vi "main OP300.2.vi"() -> ()   [LabVIEW 2020]
uses:
  SubVI/OP150ZP_state.ctl
  <userlib>/Alex.vi/FGV.ctl
  Lib/02 SLIM ZEN WS 500/SubVi/VG_progressBar.vi
  SubVI/CheminDeBase.vi
  VG/PN.vi
  VG/IS30%.vi
  SubVI/VG_HYDRAU.vi
  VG/VG_BT3562.vi
panel:
  out "error out":errorcluster
  in  "arrêt":bool
  in  "last?":bool
  out "VISA OUT 2":T1
  out "Cluster 2":T2
  out "IS30% ?":bool
  out "Cluster":T2
  out "progression":u8(slide) scale=0.0..100.0
  out "PN":string
  out "errout 2":errorcluster={"status"=TRUE, "code"=0, "source"="PCAN_CHANNEL ILLEGAL"} caption="errout"
  out "errout":errorcluster caption="sortie d'erreur"
  out "STOP":bool
  out "TOP":string
  out "DRAW":picture
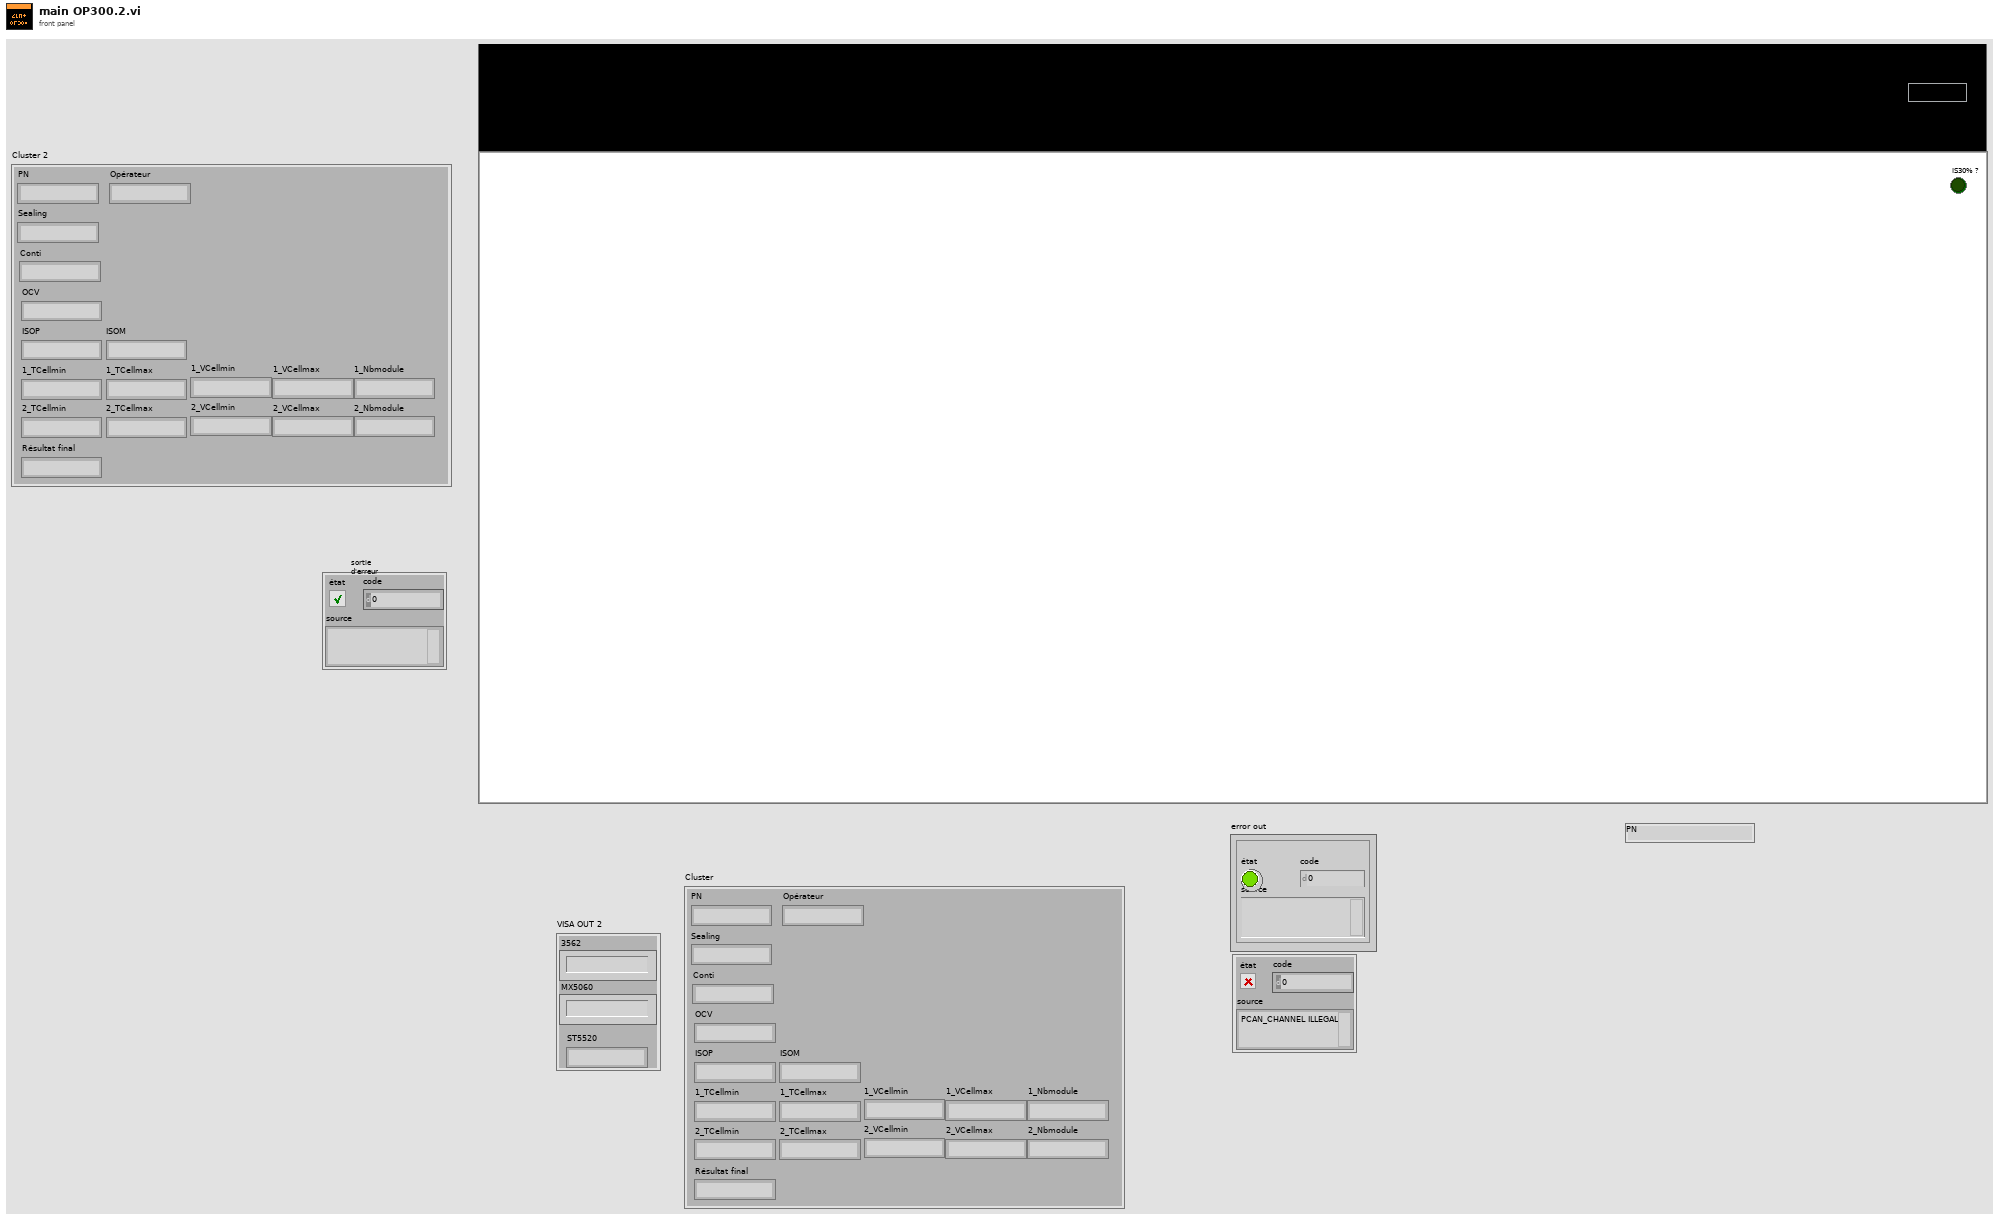
[diagram p1: front panel]
types:
  T1 = cluster{"3562":string, "MX5060":string, "ST5520":string}
  T2 = cluster{"PN":string, "Opérateur":string, "Sealing":string, "Conti":string, "OCV":string, "ISOP":string, "ISOM":string, "1_TCellmin":string, "1_TCellmax":string, "1_VCellmin":string, "1_VCellmax":string, "1_Nbmodule":string, "2_TCellmin":string, "2_TCellmax":string, "2_VCellmin":string, "2_VCellmax":string, "2_Nbmodule":string, "Résultat final":string}
  T3 = cluster{"PN":string, "Sealing":string, "Opérateur":string, "Conti":string, "OCV":string, "ISOP":string, "ISOM":string, "1_TCellmin":string, "1_TCellmax":string, "1_VCellmin":string, "1_VCellmax":string, "1_Nbmodule":string, "2_TCellmin":string, "2_TCellmax":string, "2_VCellmin":string, "2_VCellmax":string, "2_Nbmodule":string, "Résultat final":string}
  T4 = typedef "OP150ZP_state.ctl" = enum16{"Null", "Demarrage", "Init", "Scan", "Crash", "Next", "Conti", "Sealing", "Comext", ""}
  T5 = typedef "FGV.ctl" = enum16{"GET", "SET", "RAZ"}
  T6 = typedef "imagedata.ctl" = cluster{"image type":i32, "image depth":i32, "image":u8[], "mask":u8[], "colors":u32[], "Rectangle":cluster{"left":i16, "top":i16, "right":i16, "bottom":i16}}
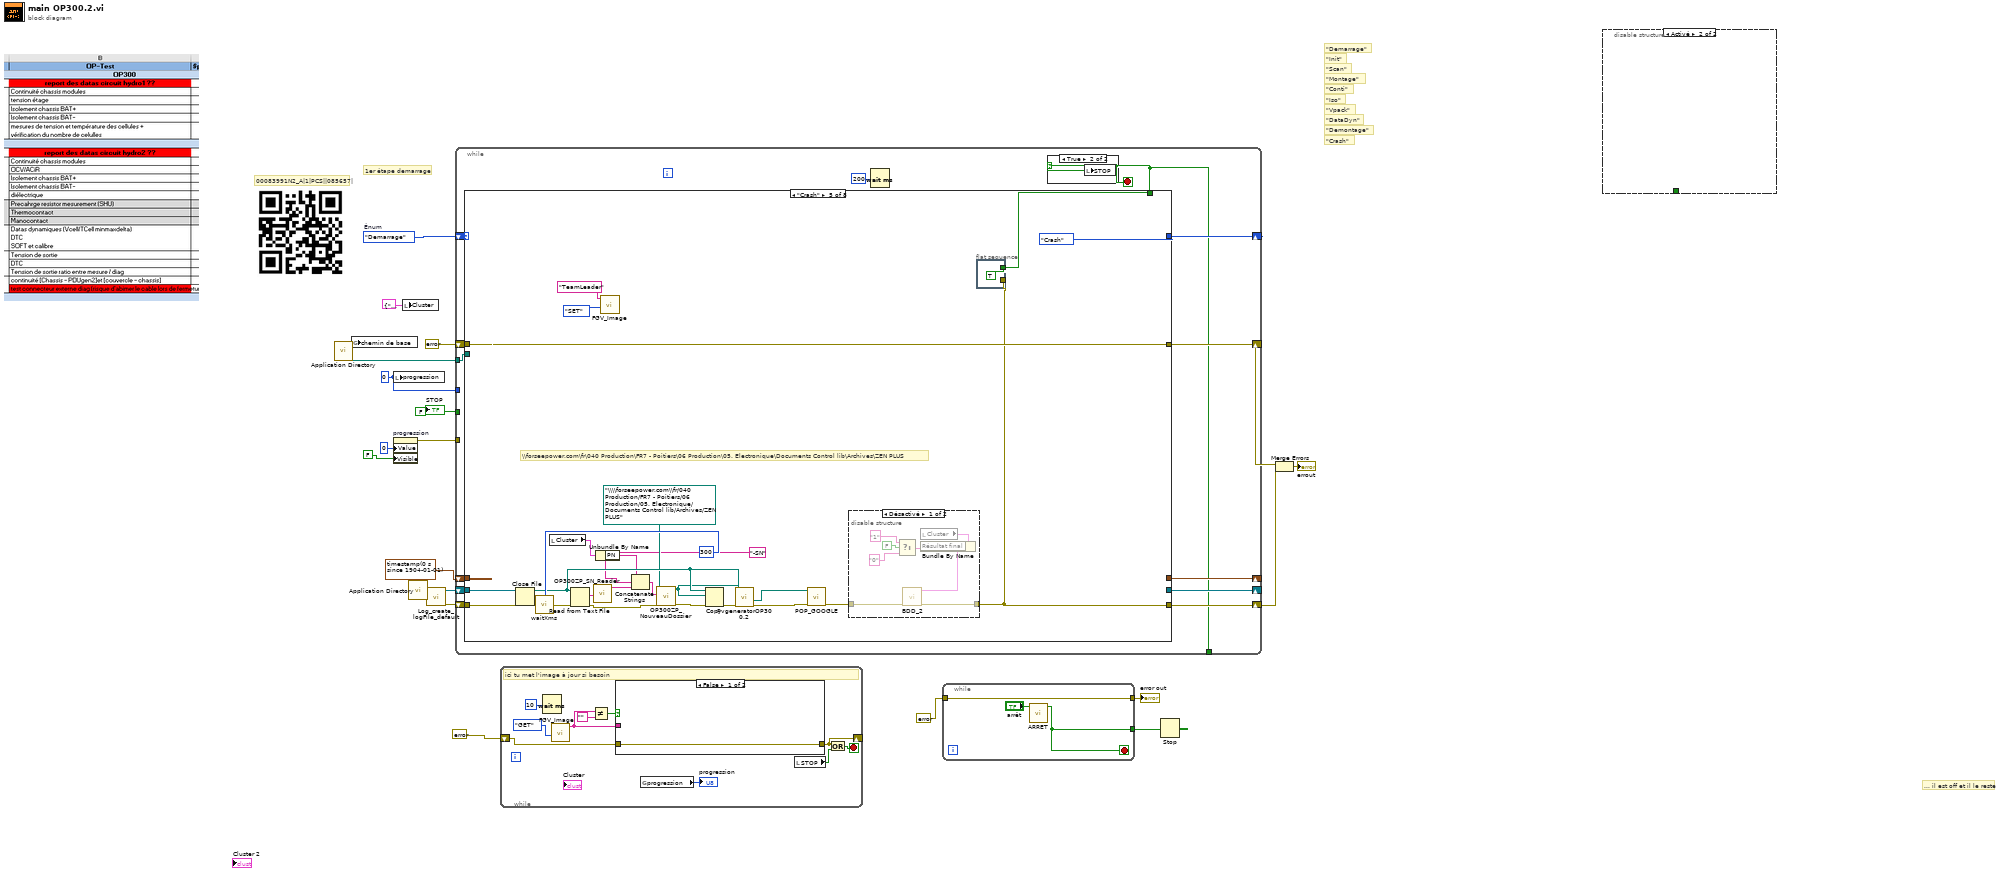
[diagram p0: block diagram]
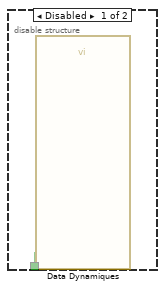
[diagram p2: hidden frame]
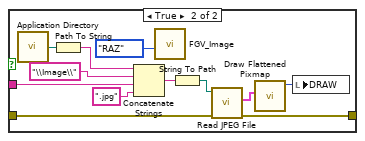
[diagram p3: hidden frame]
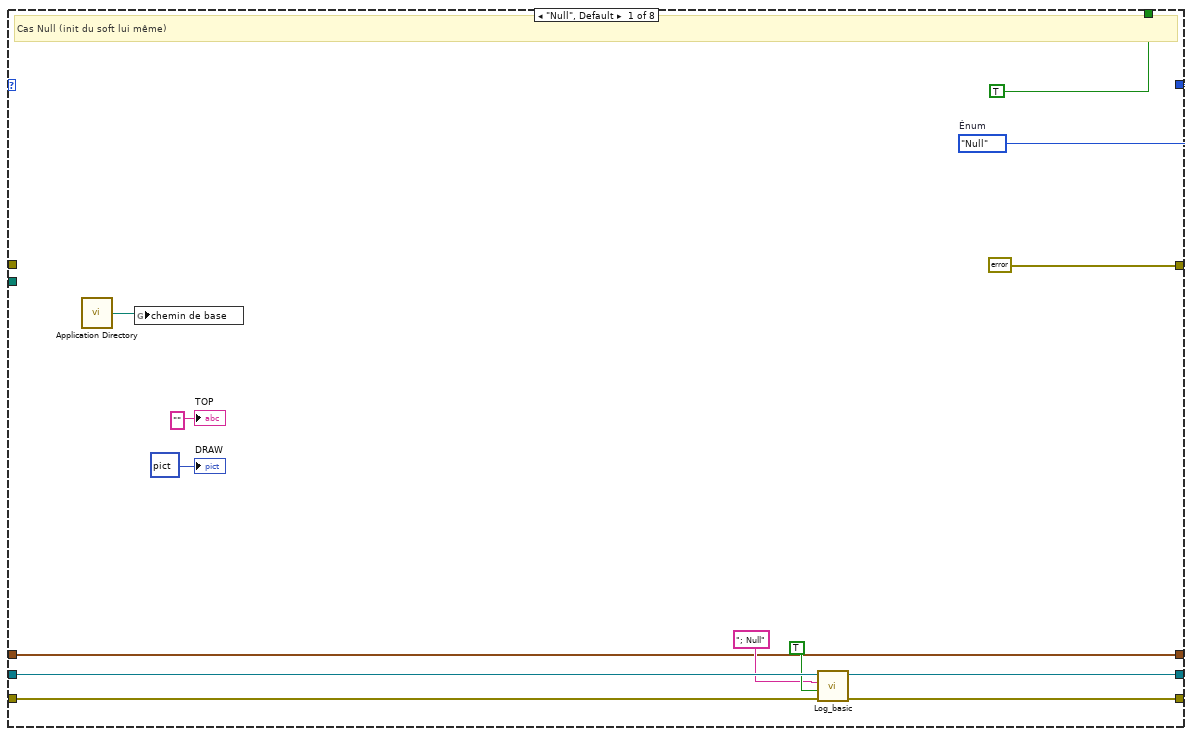
[diagram p5: hidden frame]
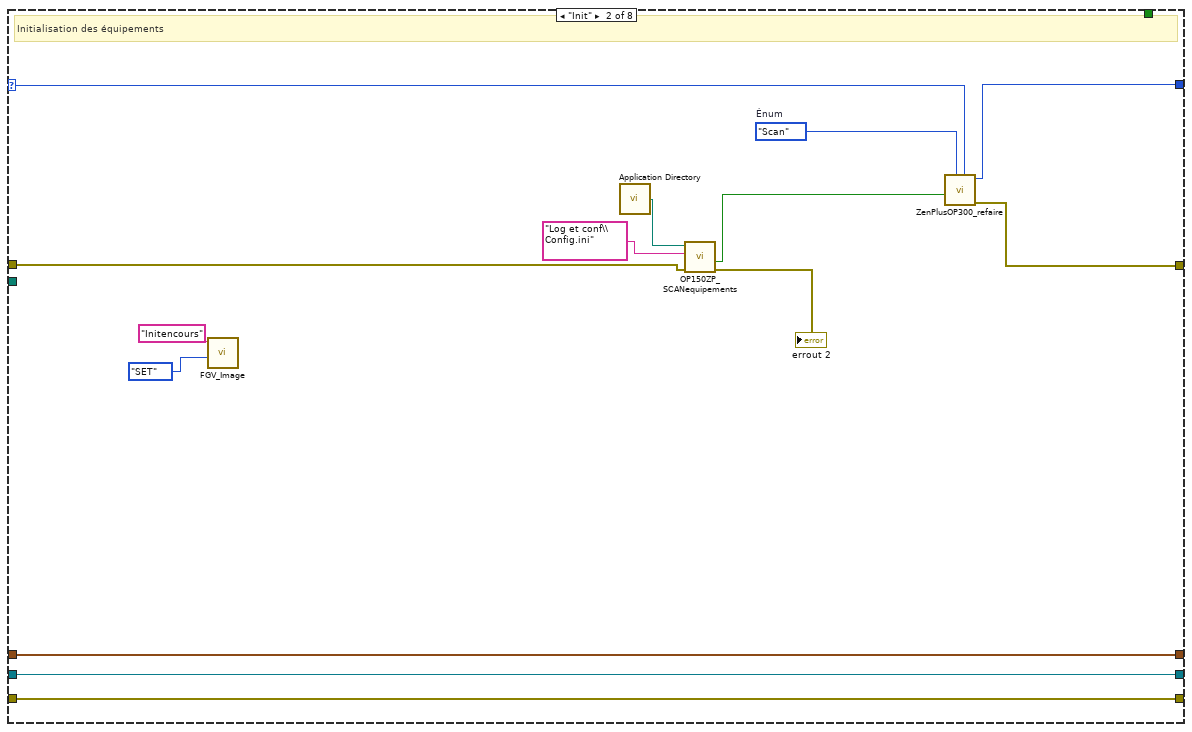
[diagram p6: hidden frame]
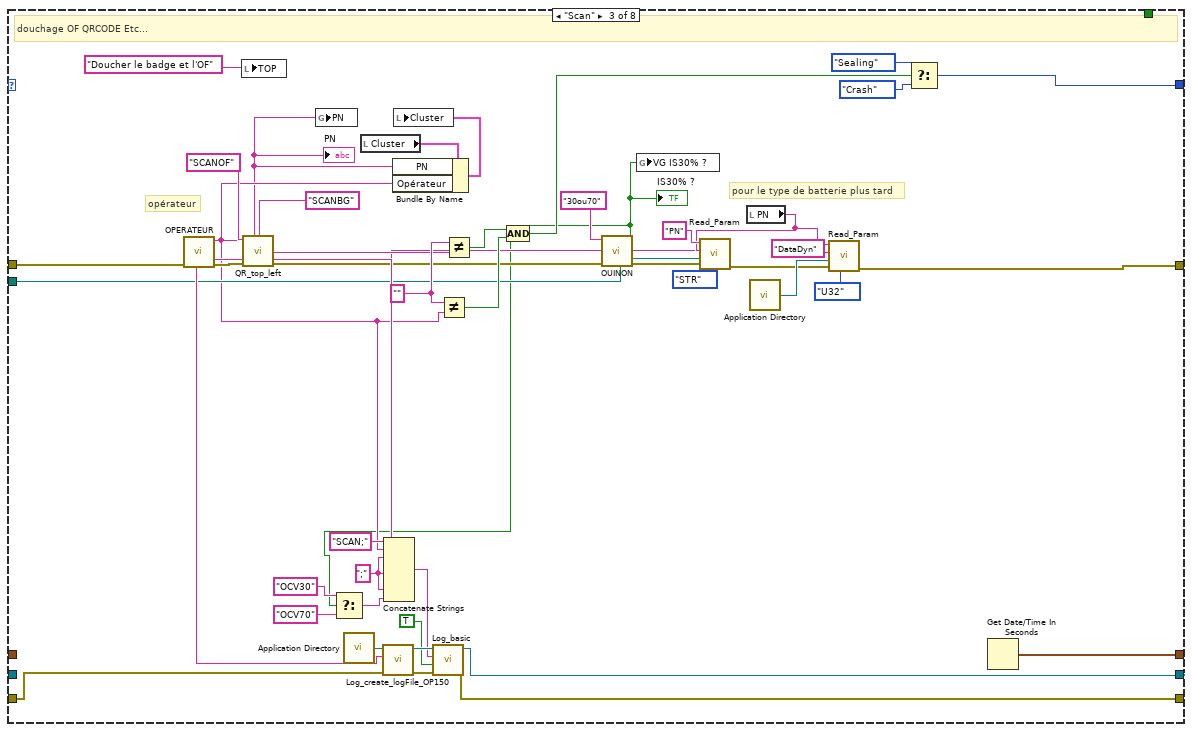
[diagram p7: hidden frame]
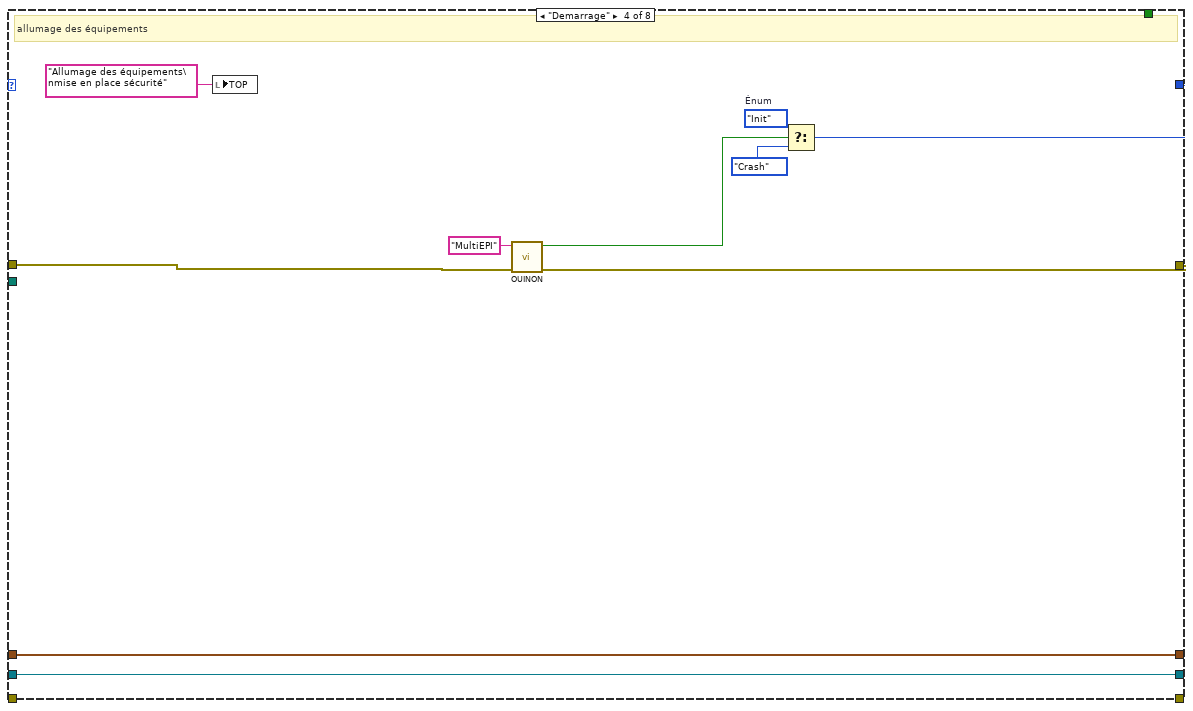
[diagram p8: hidden frame]
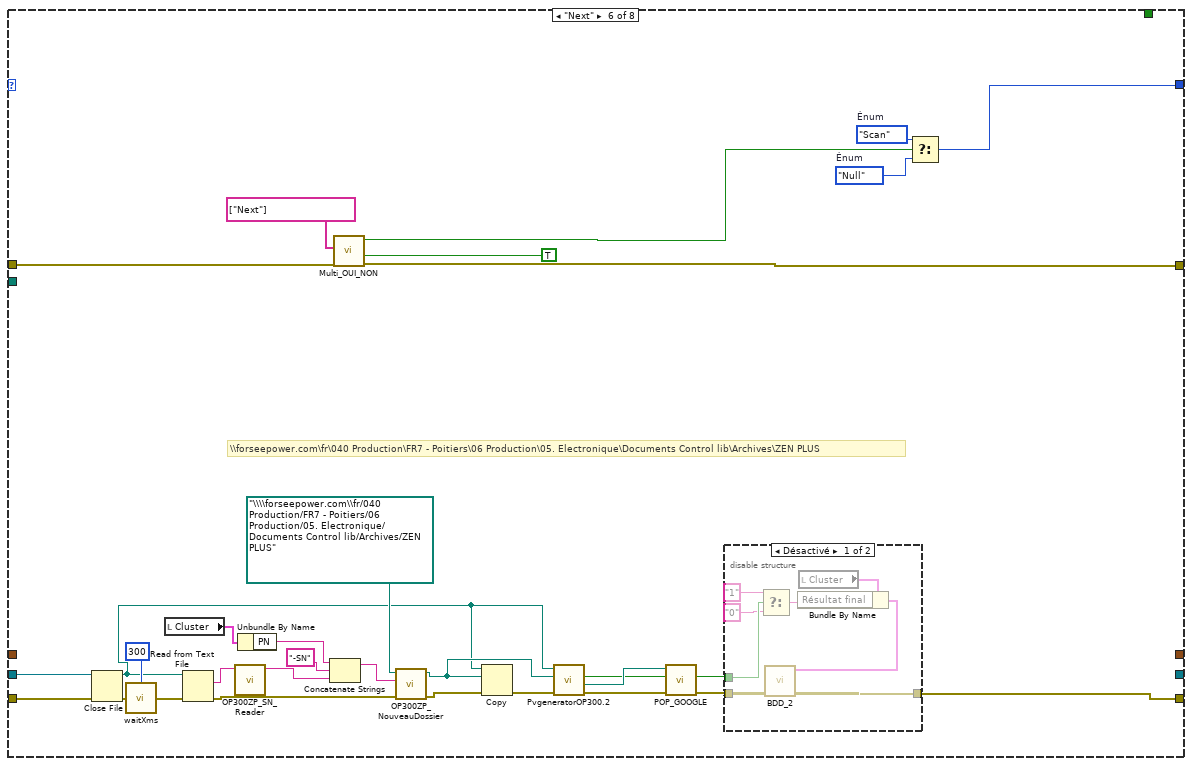
[diagram p10: hidden frame]
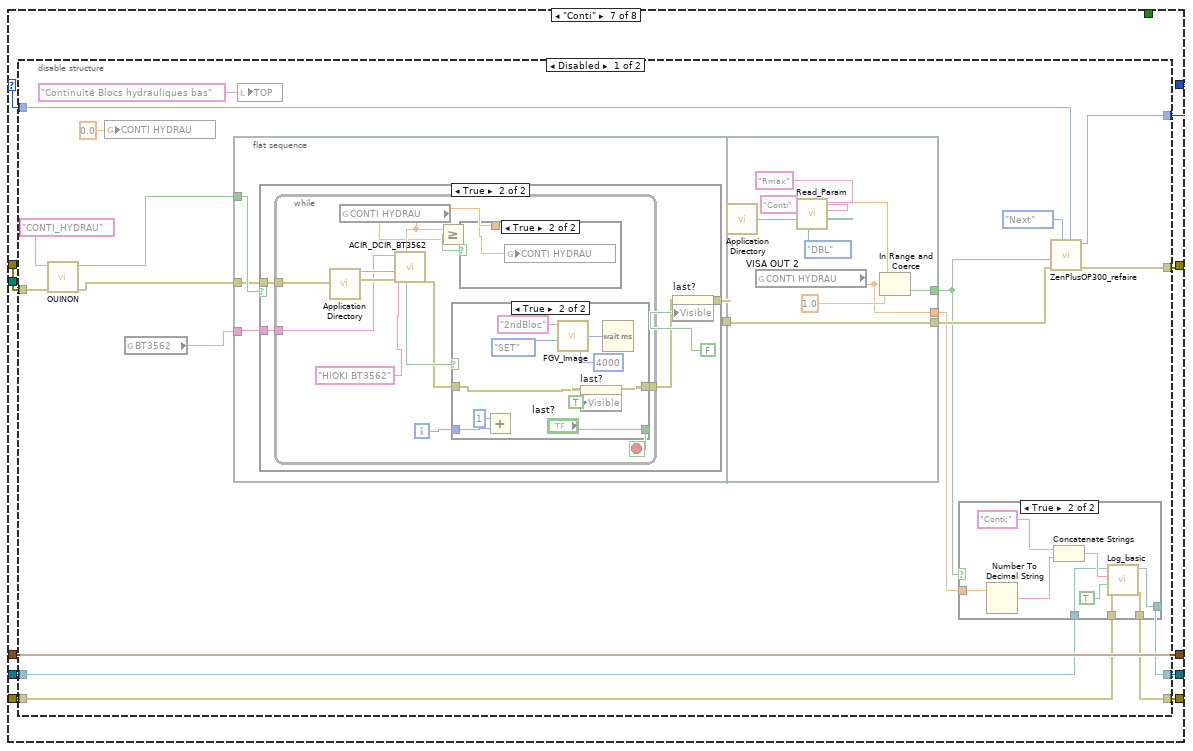
[diagram p12: hidden frame]
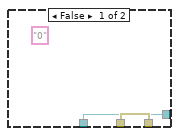
[diagram p13: hidden frame]
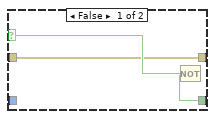
[diagram p15: hidden frame]
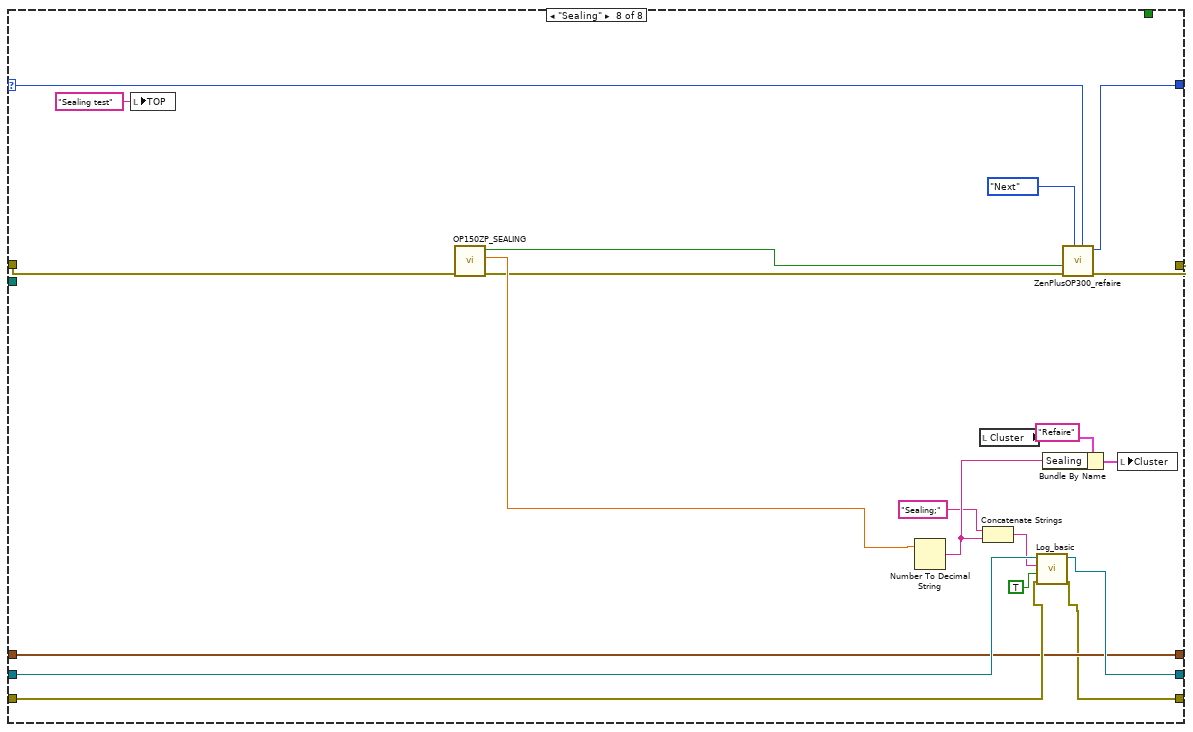
[diagram p18: hidden frame]
diagram:
  w10 = u8 0 ("progression")
  w11 = OP150ZP_state."Demarrage"  # Énum
  w17 = FALSE ("STOP")
  # "00083991N2_A|1|PCS||085657|"
  # "1er étape demarrage"
  # "\"Crash\""
  # "\"Demontage\""
  # "\"DataDyn\""
  # "\"Iso\""
  # "\"Montage\""
  # "\"Scan\""
  # "\"Init\""
  # "\"Demarrage\""
  # "\"Conti\""
  # "\"Vpack\""
  # "... il est off et il le reste"
  n1 = call <vilib>:"Application Directory.vi"() -> ("Application Directory"=w16:path)
  n2 = global write "CheminDeBase.vi" "chemin de base"(w16) -> ()
  n3 = property on="progression" class="Slide (strict)"("Value"=u8 0 ("progression"), "Visible"=FALSE) -> (error out=w8:errorcluster)  [unwired: 2 in, 1 out]
  n4 = local write "progression"(w10) -> ()
  n5 = local write "Cluster"(T3 {"PN"="0", "Sealing"="0", "Opérateur"="0", "Conti"="0", "OCV"="0", "ISOP"="0", "ISOM"="0", "1_TCellmin"="0", "1_TCellmax"="0", "1_VCellmin"="0", "1_VCellmax"="0", "1_Nbmodule"="0", "2_TCellmin"="0", "2_TCellmax"="0", "2_VCellmin"="0", "2_VCellmax"="0", "2_Nbmodule"="0", "Résultat final"="0"} ("Cluster")) -> ()
  n6 = call <vilib>:"Application Directory.vi"() -> ("Application Directory"=w14:path)
  n7 = call "Log_create_logFile_default.vi"("appdir"=w14) -> ("errout"=w15:errorcluster, "Fichier à flux d'octets en sortie"=w18:refnum<file>)  [unwired: 9 in]
  n8 = while {
    shift-right: [w32] -> w2
    shift-left: errorcluster {"status"=FALSE, "code"=0, "source"=""} ("error out") -> [w23]
    shift-right: [w22] -> _
    shift-left: w11 -> [w27]
    shift-right: [w28] -> w19
    shift-left: w15 -> [w31]
    shift-right: [w29] -> _
    shift-left: w18 -> [w30]
    tunnel: w16 -> [w26]
    tunnel: w17 -> [_]
    shift-right: [w24] -> _
    shift-left: timestamp(0 s since 1904-01-01) ("seconds since 1Jan1904") -> [w25]
    tunnel: w10 -> [_]
    tunnel: w8 -> [_]
    tunnel: [w21] -> _
    stop <- w21 stop-if-true
    n9 = case shown="\"Crash\"" w27 {
      selector: w27 -> [_ w56 _ _ _ _ w198 w282]
      tunnel: w23 -> [_ w58 w107 w109 w138 w158 w199 w280]
      tunnel: [errorcluster {"status"=FALSE, "code"=0, "source"=""} ("errin") w57 w86 w116 w138 w156 w191 w290] -> w32
      tunnel: w31 -> [w43 w61 w103 _ w141 w181 w196 w293]
      tunnel: w30 -> [w44 w60 _ w117 w142 w182 w194 w292]
      tunnel: [w41 w60 w105 w117 _ _ w193 w291] -> w29
      tunnel: [w42 w61 w106 _ w131 w174 w195 w285] -> w28
      tunnel: [TRUE _ _ _ w143 _ _ _] -> w21
      tunnel: w26 -> [_ _ w80 _ _ _ _ _]
      tunnel: w25 -> [w37 w59 _ w115 _ _ w192 w289]
      tunnel: [w37 w59 w94 w115 _ _ w192 w289] -> w24
      tunnel: [w35 w48 w62 w110 OP150ZP_state."Crash" w153 w197 w284] -> w22
      frame "Null", Default {
        w35 = OP150ZP_state."Null"  # Énum
        # "Cas Null (init du soft lui même)"
        n10 = call <vilib>:"Application Directory.vi"() -> ("Application Directory"=w47:path)
        n11 = global write "CheminDeBase.vi" "chemin de base"(w47) -> ()
        n12 = call "Log_basic.vi"("errin"=w43, "date?"=TRUE, "chaîne"="; Null", "in"=w44) -> ("sortie d'erreur"=w42:errorcluster, "refnum en sortie"=w41:refnum<file>)  [unwired: 6 in]
        "DRAW" <- picture data[5B] ("DRAW")
        "TOP" <- "" ("TOP")
      }
      frame "Init" {
        w52 = OP150ZP_state."Scan"  # Énum
        # "Initialisation des équipements"
        n13 = call <userlib>:"FGV_Image.vi"("Énum"=FGV."SET", "IN"="Initencours") -> ()  [unwired: 9 in, 1 out]
        n14 = call <vilib>:"Application Directory.vi"() -> ("Application Directory"=w49:path)
        n15 = call "OP150ZP_SCANequipements.vi"("Errin"=w58, "Chaîne"="Log et conf\\Config.ini", "pathin"=w49) -> ("ERROUT"=→"errout 2":errorcluster, "KO?"=w53:bool)  [unwired: 7 in]
        n16 = call "ZenPlusOP300_refaire.vi"("refaire"=w56, "casOK"=w52, "test ok ?"=w53) -> ("errout"=w57:errorcluster, "Next"=w48:T4)  [unwired: 7 in]
      }
      frame "Scan" {
        w66 = ";" ("chaîne")
        w97 = "" ("x")
        # "pour le type de batterie plus tard"
        # "opérateur"
        # "douchage OF QRCODE Etc..."
        n17 = call "OPERATEUR.vi"("errin"=w107, "IN"="SCANBG") -> ("error out"=w93:errorcluster, "Dataout"=w72:string)  [unwired: 8 in]
        n18 = local write "TOP"("Doucher le badge et l'OF" ("TOP")) -> ()
        n19 = call "QR_top_left.vi"("errin"=w93, "image"="SCANOF") -> ("error out"=w70:errorcluster, "Réponse"=w91:string, "SN"=w90:string, "PN"=w63:string)  [unwired: 5 in, 1 out]
        "PN" <- w63
        n20 = global write "PN.vi" "PN"(w63) -> ()
        n21 = call <vilib>:"Application Directory.vi"() -> ("Application Directory"=w104:path)
        n22 = local read "Cluster"() -> (w74:T2)
        n23 = call "Log_create_logFile_OP150.vi"("errin"=w103, "toute l'expression"=w90, "Application Directory"=w104) -> ("sortie d'erreur"=w101:errorcluster, "Fichier à flux d'octets en sortie"=w102:refnum<file>)  [unwired: 7 in]
        n24 = Bundle By Name(cluster=w74, "PN"=w63, "Opérateur"=w72) -> (w73:T2)
        n25 = local write "Cluster"(w73) -> ()
        n26 = Not Equal?(x=w97, y=w72) -> (x != y?=w95:bool)
        n27 = Not Equal?(x=w97, y=w91) -> (x != y?=w96:bool)
        n28 = Compound Arithmetic op=AND ("Opérateur arithmétique")(w96, w95) -> (w78:bool)
        n29 = call "OUINON.vi"("errin"=w70, "image"="30ou70") -> ("error out"=w69:errorcluster, "OUI/NON"=w64:bool)  [unwired: 8 in]
        "IS30% ?" <- w64
        n30 = Select ("Sélectionner")(t="OCV30" ("section"), s=w64, f="OCV70" ("section")) -> (s? t:f=w65:string)
        n31 = global write "IS30%.vi" "VG IS30% ?"(w64) -> ()
        n32 = local read "PN"() -> (w82:string)
        n33 = call "Read_Param.vi"("Énum"=enum16{"STR", "DBL", "U32"}."STR", "errin"=w69, "pathin"=w80, "section"=w82, "key"="PN") -> ("error out"=w85:errorcluster, "str"=w81:string)  [unwired: 2 in, 3 out]
        n34 = Concatenate Strings("SCAN;" ("chaîne"), w72, w66, w90, w66, w81, w66, w65) -> (w99:string)
        n35 = call "Log_basic.vi"("errin"=w101, "date?"=TRUE, "chaîne"=w99, "in"=w102) -> ("sortie d'erreur"=w106:errorcluster, "refnum en sortie"=w105:refnum<file>)  [unwired: 6 in]
        n36 = call <vilib>:"Application Directory.vi"() -> ("Application Directory"=w89:path)
        n37 = call "Read_Param.vi"("Énum"=enum16{"STR", "DBL", "U32"}."U32", "errin"=w85, "pathin"=w89, "section"="DataDyn", "key"=w82) -> ("error out"=w86:errorcluster)  [unwired: 2 in, 4 out]
        n38 = Select ("Sélectionner")(t=OP150ZP_state."Sealing" ("Énum"), s=w78, f=OP150ZP_state."Crash" ("cas faux")) -> (s? t:f=w62:T4)
        n39 = Get Date/Time In Seconds() -> (seconds since 1Jan1904=w94:timestamp)
      }
      frame "Demarrage" {
        w112 = OP150ZP_state."Init"  # Énum
        # "allumage des équipements"
        n40 = local write "TOP"("Allumage des équipements\nmise en place sécurité" ("TOP")) -> ()
        n41 = call "OUINON.vi"("errin"=w109, "image"="MultiEPI" ("IN")) -> ("error out"=w116:errorcluster, "OUI/NON"=w113:bool)  [unwired: 8 in]
        n42 = Select ("Sélectionner")(t=w112, s=w113, f=OP150ZP_state."Crash" ("cas faux")) -> (s? t:f=w110:T4)
      }
      frame "Crash" {
        # "\\\\forseepower.com\\fr\\040 Production\\FR7 - Poitiers\\06 Production\\05. Electronique\\Documents Control lib\\Archives\\ZEN PLUS"
        n43 = Close File(refnum=w142, error in=w141) -> (path=w129:path, error out=w134:errorcluster)
        n44 = call <userlib>:"waitXms.vi"("attente (ms)"=u32 300, "errin"=w134) -> ("errout"=w130:errorcluster)  [unwired: 13 in]
        n45 = local read "Cluster"() -> (w123:T2)
        n46 = Read from Text File(file (use dialog)=w129, error in=w130) -> (text=w128:string, error out=w126:errorcluster)  [unwired: 2 in, 2 out]
        n47 = call "OP300ZP_SN_Reader.vi"("Fichier txt"=w128) -> ("SN"=w121:string)  [unwired: 10 in]
        n48 = Unbundle By Name(w123) -> ("PN"=w120:string)
        n49 = call <userlib>:"FGV_Image.vi"("Énum"=FGV."SET", "IN"="TeamLeader") -> ()  [unwired: 9 in, 1 out]
        n50 = Concatenate Strings(w120, "-SN" ("chaîne"), w121) -> (w122:string)
        n51 = call "OP300ZP_NouveauDossier.vi"("entrée d'erreur (pas d'erreur)"=w126, "Nom du repertoire (PN SN)"=w122, "Network before adding a new folder"=path "\\\\forseepower.com\\fr/040 Production/FR7 - Poitiers/06 Production/05. Electronique/Documents Control lib/Archives/ZEN PLUS" ("chemin de la cible (utiliser une boîte de dialogue)")) -> ("sortie d'erreur"=w127:errorcluster, "Network after adding a new folder"=w124:path)  [unwired: 7 in]
        n52 = Copy ("Copier")(8:w127, 10:w124, 11:w129) -> (0:w133:errorcluster)  [unwired: 2 in, 2 out]
        n53 = call "PvgeneratorOP300.2.vi"("errin"=w133, "network"=w124, "path in"=w129) -> ("sortie d'erreur"=w137:errorcluster, "network out"=w136:path)  [unwired: 5 in, 2 out]
        n54 = call "POP_GOOGLE.vi"("error in"=w137, "chemin"=w136) -> ("error out"=w132:errorcluster)  [unwired: 8 in, 1 out]
        n55 = disable-structure shown="Désactivé" {
          disable-tunnel: w132 -> [w151 _]
          disable-tunnel: [w150 _] -> w131
          frame Disabled {
            n56 = Select ("Sélectionner")(t="1", s=FALSE ("sélecteur"), f="0" ("cas faux")) -> (s? t:f=w146:string)
            n57 = local read "Cluster"() -> (w149:T2)
            n58 = Bundle By Name(cluster=w149, "Résultat final"=w146) -> (w145:T2)
            n59 = call "BDD_2.vi"("errin"=w151, "Cluster"=w145) -> ("error out"=w150:errorcluster)  [unwired: 8 in, 1 out]
          }
          frame Enabled {
          }
        }
        n60 = flat-sequence {
          tunnel: [TRUE] -> w143
          tunnel: w131 -> [_]
          frame #0 {
          }
        }
      }
      frame "Next" {
        w179 = OP150ZP_state."Null"  # Énum
        w180 = OP150ZP_state."Scan"  # Énum
        # "\\\\forseepower.com\\fr\\040 Production\\FR7 - Poitiers\\06 Production\\05. Electronique\\Documents Control lib\\Archives\\ZEN PLUS"
        n61 = Close File(refnum=w182, error in=w181) -> (path=w159:path, error out=w178:errorcluster)
        n62 = call <userlib>:"waitXms.vi"("attente (ms)"=u32 300, "errin"=w178) -> ("errout"=w171:errorcluster)  [unwired: 13 in]
        n63 = local read "Cluster"() -> (w164:T2)
        n64 = Read from Text File(file (use dialog)=w159, error in=w171) -> (text=w169:string, error out=w168:errorcluster)  [unwired: 2 in, 2 out]
        n65 = call "OP300ZP_SN_Reader.vi"("Fichier txt"=w169) -> ("SN"=w161:string)  [unwired: 10 in]
        n66 = Unbundle By Name(w164) -> ("PN"=w163:string)
        n67 = Concatenate Strings(w163, "-SN" ("chaîne"), w161) -> (w160:string)
        n68 = call "Multi_OUI_NON.vi"("errin"=w158, "errinb"=TRUE, "Tableau"=string[] ["Next"]) -> ("errout"=w156:errorcluster, "isok?"=w155:bool)  [unwired: 7 in]
        n69 = call "OP300ZP_NouveauDossier.vi"("entrée d'erreur (pas d'erreur)"=w168, "Nom du repertoire (PN SN)"=w160, "Network before adding a new folder"=path "\\\\forseepower.com\\fr/040 Production/FR7 - Poitiers/06 Production/05. Electronique/Documents Control lib/Archives/ZEN PLUS" ("chemin de la cible (utiliser une boîte de dialogue)")) -> ("sortie d'erreur"=w167:errorcluster, "Network after adding a new folder"=w165:path)  [unwired: 7 in]
        n70 = Copy ("Copier")(8:w167, 10:w165, 11:w159) -> (0:w170:errorcluster)  [unwired: 2 in, 2 out]
        n71 = call "PvgeneratorOP300.2.vi"("errin"=w170, "network"=w165, "path in"=w159) -> ("sortie d'erreur"=w176:errorcluster, "network out"=w175:path, "tout bon"=w172:bool)  [unwired: 5 in, 1 out]
        n72 = call "POP_GOOGLE.vi"("error in"=w176, "chemin"=w175) -> ("error out"=w173:errorcluster)  [unwired: 8 in, 1 out]
        n73 = disable-structure shown="Désactivé" {
          disable-tunnel: [w190 _] -> w174
          disable-tunnel: w173 -> [w189 _]
          disable-tunnel: w172 -> [w187 _]
          frame Disabled {
            n74 = Select ("Sélectionner")(t="1", s=w187, f="0" ("cas faux")) -> (s? t:f=w184:string)
            n75 = local read "Cluster"() -> (w188:T2)
            n76 = Bundle By Name(cluster=w188, "Résultat final"=w184) -> (w183:T2)
            n77 = call "BDD_2.vi"("errin"=w189, "Cluster"=w183) -> ("error out"=w190:errorcluster)  [unwired: 8 in, 1 out]
          }
          frame Enabled {
          }
        }
        n78 = Select(t=w180, s=w155, f=w179) -> (s? t:f=w153:T4)
      }
      frame "Conti" {
        n79 = disable-structure shown="Disabled" {
          disable-tunnel: w199 -> [w217 _]
          disable-tunnel: w198 -> [w216 _]
          disable-tunnel: [w215 _] -> w197
          disable-tunnel: w196 -> [w214 _]
          disable-tunnel: [w213 _] -> w195
          disable-tunnel: w194 -> [w212 _]
          disable-tunnel: [w211 _] -> w193
          disable-tunnel: [w210 _] -> w191
          frame Disabled {
            n80 = call "OUINON.vi"("errin"=w217, "image"="CONTI_HYDRAU" ("IN")) -> ("error out"=w201:errorcluster, "OUI/NON"=w206:bool)  [unwired: 8 in]
            n81 = global write "VG_HYDRAU.vi" "CONTI HYDRAU"(0.0 ("R")) -> ()
            n82 = global read "VG_BT3562.vi" "BT3562"() -> (w200:string)
            n83 = flat-sequence {
              tunnel: w206 -> [w233]
              tunnel: w200 -> [w232]
              tunnel: w201 -> [w231]
              tunnel: [w230] -> w218
              tunnel: [w267] -> w202
              tunnel: [w266] -> w203
              tunnel: [w265] -> w204
              tunnel: w218 -> [w265]
              frame #0 {
                n84 = case shown="True" w233 {
                  tunnel: w232 -> [_ w239]
                  tunnel: w231 -> [w234 w238]
                  tunnel: [w234 w236] -> w230
                  frame False {
                  }
                  frame True {
                    n85 = while {
                      tunnel: w239 -> [w241]
                      tunnel: w238 -> [w251]
                      tunnel: [w248] -> w235
                      i -> [w247]
                      stop <- w244 stop-if-true
                      n86 = call <vilib>:"Application Directory.vi"() -> ("Application Directory"=w250:path)
                      n87 = global read "VG_HYDRAU.vi" "CONTI HYDRAU"() -> (w242:dbl)
                      n88 = call <instrlib>:"ACIR_DCIR_BT3562.vi"("errin"=w251, "chemin de base"=w250, "section"="HIOKI BT3562", "VISAin"=w241) -> ("errout"=w243:errorcluster, "OK?"=w249:bool, "R"=w245:dbl)  [unwired: 1 in, 4 out]
                      n89 = Greater Or Equal?(x=w245, y=w242) -> (x >= y?=w246:bool)
                      n90 = case shown="True" w249 {
                        selector: w249 -> [w254 _]
                        tunnel: w243 -> [w252 w256]
                        tunnel: [w252 w258] -> w248
                        tunnel: [w253 "last?"] -> w244
                        tunnel: w247 -> [_ w261]
                        frame False {
                          n91 = Not(x=w254) -> (.not. x?=w253:bool)
                        }
                        frame True {
                          n92 = Add(x=1, y=w261) -> ()  [unwired: 1 out]
                          n93 = call <userlib>:"FGV_Image.vi"("Énum"=FGV."SET", "IN"="2ndBloc") -> ()  [unwired: 9 in, 1 out]
                          n94 = property on="last?" class="Bool"(error in=w256, "Visible"=TRUE) -> (error out=w258:errorcluster)  [unwired: 1 in, 1 out]
                          n95 = Wait (ms)(milliseconds to wait=u32 4000 ("attente (ms)")) -> ()  [unwired: 1 out]
                        }
                      }
                      n96 = case shown="True" w246 {
                        tunnel: w245 -> [_ w264]
                        frame False {
                        }
                        frame True {
                          n97 = global write "VG_HYDRAU.vi" "CONTI HYDRAU"(w264) -> ()
                        }
                      }
                    }
                    n98 = property on="last?" class="Bool"(error in=w235, "Visible"=FALSE) -> (error out=w236:errorcluster)  [unwired: 1 in, 1 out]
                  }
                }
              }
              frame #1 {
                n99 = call <vilib>:"Application Directory.vi"() -> ("Application Directory"=w271:path)
                n100 = global read "VG_HYDRAU.vi" "CONTI HYDRAU"() -> (w266:dbl)
                n101 = call "Read_Param.vi"("Énum"=enum16{"STR", "DBL", "U32"}."DBL", "pathin"=w271, "section"="Conti", "key"="Rmax") -> ("dbl"=w269:dbl)  [unwired: 3 in, 4 out]
                n102 = In Range and Coerce(upper limit=w269, x=w266, lower limit=1.0 ("limite inférieure")) -> (In Range?=w267:bool)  [unwired: 1 out]
              }
            }
            n103 = local write "TOP"("Continuité Blocs hydrauliques bas" ("TOP")) -> ()
            n104 = case shown="True" w202 {
              tunnel: [w219 w227] -> w211
              tunnel: [w220 w226] -> w213
              tunnel: w203 -> [_ w225]
              tunnel: w214 -> [w220 w223]
              tunnel: w212 -> [w219 w222]
              frame False {
                (unwired) "0"
              }
              frame True {
                n105 = Number To Decimal String(number=w225) -> (decimal integer string=w221:string)  [unwired: 1 in]
                n106 = Concatenate Strings("Conti;" ("chaîne"), w221) -> (w228:string)
                n107 = call "Log_basic.vi"("errin"=w223, "date?"=TRUE, "chaîne"=w228, "in"=w222) -> ("sortie d'erreur"=w226:errorcluster, "refnum en sortie"=w227:refnum<file>)  [unwired: 6 in]
              }
            }
            n108 = call "ZenPlusOP300_refaire.vi"("refaire"=w216, "casOK"=OP150ZP_state."Next" ("refaire"), "errin"=w204, "test ok ?"=w202) -> ("errout"=w210:errorcluster, "Next"=w215:T4)  [unwired: 6 in]
          }
          frame Enabled {
          }
        }
      }
      frame "Sealing" {
        (unwired) "Refaire" ("image")
        n109 = local write "TOP"("Sealing test" ("TOP")) -> ()
        n110 = call "OP150ZP_SEALING.vi"("ERRIN"=w280) -> ("ERROUT"=w274:errorcluster, "SEALING_VALUE"=w279:dbl, "IsOK?"=w275:bool)  [unwired: 8 in]
        n111 = Number To Decimal String(number=w279) -> (decimal integer string=w286:string)  [unwired: 1 in]
        n112 = local read "Cluster"() -> (w288:T2)
        n113 = Concatenate Strings("Sealing;" ("chaîne"), w286) -> (w277:string)
        n114 = call "Log_basic.vi"("errin"=w293, "date?"=TRUE, "chaîne"=w277, "in"=w292) -> ("sortie d'erreur"=w285:errorcluster, "refnum en sortie"=w291:refnum<file>)  [unwired: 6 in]
        n115 = Bundle By Name(cluster=w288, "Sealing"=w286) -> (w287:T2)
        n116 = call "ZenPlusOP300_refaire.vi"("refaire"=w282, "casOK"=OP150ZP_state."Next" ("refaire"), "errin"=w274, "test ok ?"=w275) -> ("errout"=w290:errorcluster, "Next"=w284:T4)  [unwired: 6 in]
        n117 = local write "Cluster"(w287) -> ()
      }
    }
    n118 = Wait (ms)(milliseconds to wait=u32 200 ("attente (ms)")) -> ()  [unwired: 1 out]
    n119 = case shown="True" w21 {
      selector: w21 -> [_ w34]
      frame False {
      }
      frame True {
        n120 = local write "STOP"(w34) -> ()
      }
    }
  }
  n121 = while {
    shift-right: [w302] -> _
    shift-left: errorcluster {"status"=FALSE, "code"=0, "source"=""} ("error out") -> [w299]
    stop <- w300 stop-if-true
    # "ici tu met l'image à jour si besoin"
    n122 = Wait (ms)(milliseconds to wait=u32 10 ("attente (ms)")) -> ()  [unwired: 1 out]
    n123 = call <userlib>:"FGV_Image.vi"("Énum"=FGV."GET") -> ("OUT"=w295:string)  [unwired: 10 in]
    n124 = Not Equal?(x=w295, y="") -> (x != y?=w296:bool)
    n125 = case shown="False" w296 {
      tunnel: [w304 w309] -> w302
      tunnel: w299 -> [w304 w308]
      tunnel: w295 -> [_ w307]
      frame False {
      }
      frame True {
        n126 = call <vilib>:"Application Directory.vi"() -> ("Application Directory"=w312:path)
        n127 = Path To String(path=w312) -> (string=w313:string)
        n128 = Concatenate Strings(w313, "\\Image\\" ("chaîne"), w307, ".jpg" ("chaîne")) -> (w311:string)
        n129 = call <userlib>:"FGV_Image.vi"("Énum"=FGV."RAZ") -> ()  [unwired: 10 in, 1 out]
        n130 = String To Path(string=w311) -> (path=w310:path)
        n131 = call <vilib>:"Read JPEG File.vi"("error in (no error)"=w308, "path to JPEG file"=w310) -> ("error out"=w309:errorcluster, "image data"=w316:T6)  [unwired: 7 in, 1 out]
        n132 = call <vilib>:"Draw Flattened Pixmap.vi"("image data"=w316) -> ("new picture"=w305:picture)  [unwired: 8 in]
        n133 = local write "DRAW"(w305) -> ()
      }
    }
    n134 = global read "VG_progressBar.vi" "progression"() -> (→"progression":u8)
    n135 = local read "STOP"() -> (w301:bool)
    n136 = Or(x=w302, y=w301) -> (x .or. y?=w300:bool)
  }
  n137 = while {
    tunnel: [w318] -> w3
    tunnel: errorcluster {"status"=FALSE, "code"=0, "source"=""} ("error out") -> [w318]
    tunnel: [w317] -> w1
    stop <- w317 stop-if-true
    n138 = call <userlib>:"ARRET.vi"("arrêt"="arrêt") -> ("T button?"=w317:bool)  [unwired: 10 in]
  }
  "error out" <- w3
  n139 = Stop(stop? (T)=w1) -> ()
  n140 = Merge Errors(w2, w19) -> (→"errout":errorcluster)
  n141 = disable-structure shown="Activé" {
    disable-tunnel: [w320 _] -> _
    frame Disabled {
      n142 = call "Data Dynamiques"() -> ("CMU OK"=w320:bool)  [unwired: 12 in, 7 out]
    }
    frame Enabled {
    }
  }
  "STOP" <- w17
